vi "Open Spreadsheet Core.vi"(8 "error in (no error)":errorcluster, 10 "FileStream":refnum<k24>, 11 "Excel Legacy in":refnum<class "Excel Legacy.lvclass">) -> (0 "error out":errorcluster, 3 "Excel Legacy out":refnum<class "Excel Legacy.lvclass">)   [LabVIEW 2013, in "Excel Legacy.lvclass"]
uses:
  Excel Legacy.lvclass
  C:/PhaeronGit/LVNPOI/Resources/NPOI 2.1.1 dotnet2/NPOI.dll
  Resources/NPOI 2.1.1 dotnet2/NPOI.dll
  Excel Legacy.lvclass/Excel Legacy.ctl
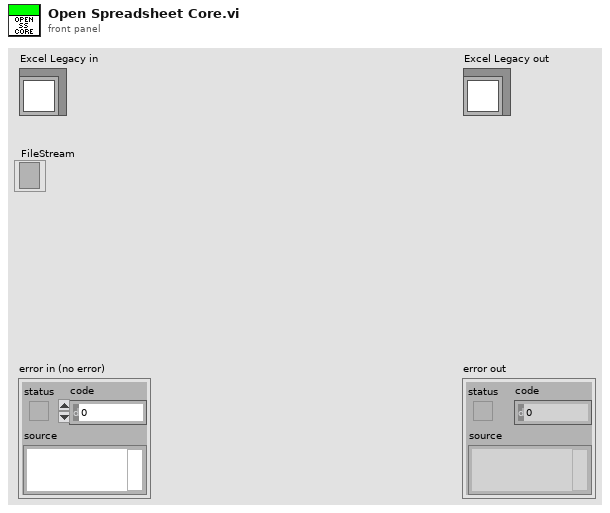
[diagram p1: front panel]
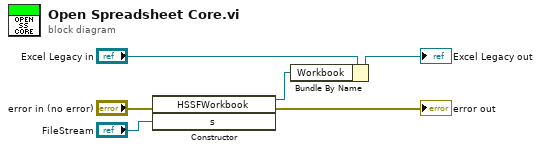
[diagram p0: block diagram]
diagram:
  n1 = constructor class="HSSFWorkbook"(error in="error in (no error)", "s"="FileStream") -> (reference out=w2:refnum<k24>, error out=→"error out":errorcluster)  [unwired: 2 in, 2 out]
  n2 = Bundle By Name(cluster="Excel Legacy in", "Workbook"=w2) -> (→"Excel Legacy out":refnum<class "Excel Legacy.lvclass">)
